vi "CSTK_Icon_Creator_CreateLogo_InputPath.vi"(8 "错误输入（无错误）":errorcluster) -> (0 "错误输出":errorcluster, 2 "OK?":bool, 3 "文件夹路径输出":path)   [LabVIEW 2015, in "CSTK_Icon Creator.lvlib"]
uses:
  CSTK_Icon Creator.lvlib
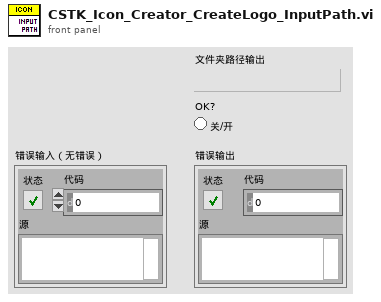
[diagram p1: front panel]
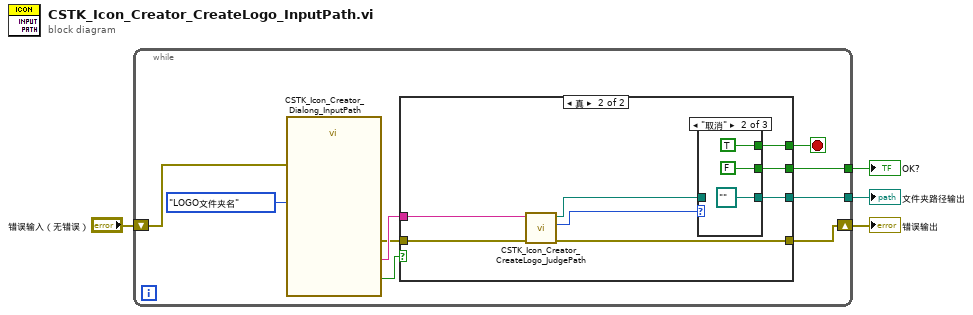
[diagram p0: block diagram]
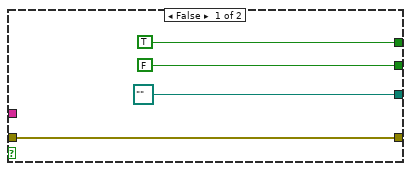
[diagram p2: hidden frame]
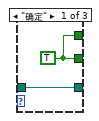
[diagram p3: hidden frame]
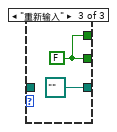
[diagram p4: hidden frame]
diagram:
  n1 = while {
    shift-right: [w12] -> w4
    shift-left: "错误输入（无错误）" -> [w9]
    tunnel: [w6] -> w2
    tunnel: [w5] -> w1
    stop <- w7 stop-if-true
    n2 = call "CSTK_Icon_Creator_Dialong_InputPath.vi"("error in (no error)"=w9, "名称"=enum16{"分类文件夹名", "LOGO文件夹名"}."LOGO文件夹名") -> ("分类文件夹名输出"=w13:string, "确定"=w8:bool, "error out"=w11:errorcluster)  [unwired: 15 in]
    n3 = case shown="真" w8 {
      tunnel: w13 -> [_ w25]
      tunnel: [w15 w24] -> w12
      tunnel: w11 -> [w15 w23]
      tunnel: [TRUE w18] -> w7
      tunnel: [path "" w20] -> w6
      tunnel: [FALSE w19] -> w5
      frame False {
      }
      frame True {
        n4 = call "CSTK_Icon_Creator_CreateLogo_JudgePath.vi"("error in"=w23, "文件夹名输入"=w25) -> ("error out"=w24:errorcluster, "result"=w22:enum16{"确定", "取消", "重新输入"}, "文件夹路径输出"=w21:path)  [unwired: 7 in]
        n5 = case shown="\"取消\"" w22 {
          tunnel: [w27 path "" path ""] -> w20
          tunnel: w21 -> [w27 _ _]
          tunnel: [w26 FALSE w32] -> w19
          tunnel: [w26 TRUE w32] -> w18
          frame "确定" {
            w26 = TRUE
          }
          frame "取消" {
          }
          frame "重新输入" {
            w32 = FALSE
          }
        }
      }
    }
  }
  "错误输出" <- w4
  "文件夹路径输出" <- w2
  "OK?" <- w1
